vi "VariableManager.vi"() -> (3 "VariableManager":refnum<class "VariableManager.lvclass">)   [LabVIEW 2013, in "VariableManagerAPI.lvlib"]
doc: "Return VariableManager object.\nData can be accessed through property node.\n\n<B>Semaphore</B>: the internal semaphore for synchronized access to the object through reference.\n<B>Variables</B>: the array of variable definition\n<B>SequenceIndices</B>: the array of sequence index definition\n<B>VariableGroups</B>: the array of VariableGroup\n<B>UpdateEvent</B>: the internal user event for values changes in VariableManager\n<B>UpdatedValues</B>: the internal boolean for variable values evaluation\n<B>SequenceValues</B>: the evaluated sequenced variable value\n<B>DefaultValues</B>: the evaluated default variable value\n<B>LastAcquireValues</B>: the variable values from the last call of GetVariableValues.vi"
uses:
  VariableManagerAPI.lvlib
  VariableManager/VariableManager.lvclass
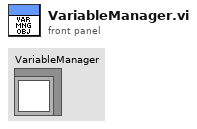
[diagram p1: front panel]
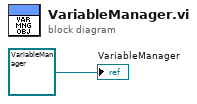
[diagram p0: block diagram]
diagram:
  "VariableManager" <- refnum<class "VariableManager.lvclass"> refnum ("VariableManager.lvclass")
